vi "FTW-Message-Request-Interpret.vi"(8 "error in":errorcluster, 11 "FTW Incoming Request":refnum<class "FTW-Message-IncomingRequest.lvclass">) -> (0 "error out":errorcluster, 1 "Request Body":string, 2 "Request Header":string, 3 "FTW Incoming Request out":refnum<class "FTW-Message-IncomingRequest.lvclass">, 4 "Request Metadata":string)   [LabVIEW 2013, in "FTW-Message-IncomingRequest.lvclass"]
uses:
  FTW-Message-IncomingRequest.lvclass
  Base/FTW-Message.lvclass
panel:
  # "Inputs"
  # "Outputs"
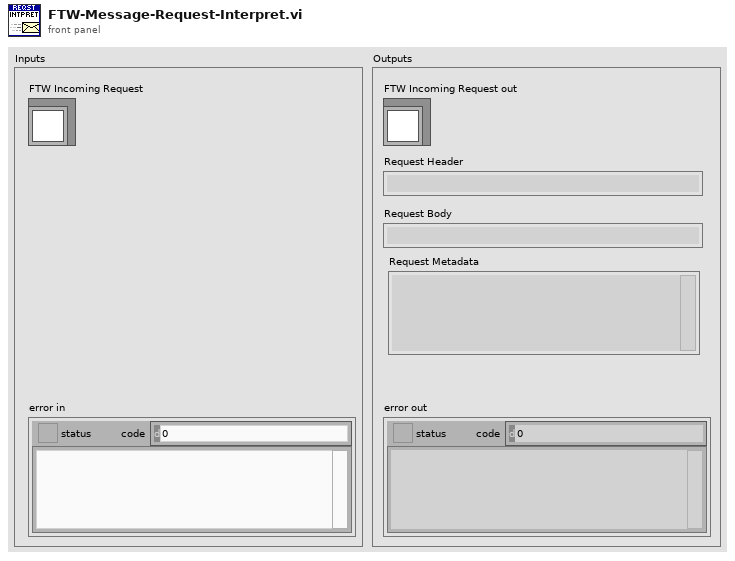
[diagram p1: front panel]
types:
  T1 = typedef "FTW-MessagePayload.ctl" = cluster{"Header":string, "Body":string, "Metadata":string}
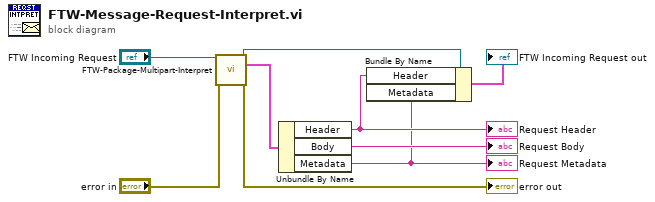
[diagram p0: block diagram]
diagram:
  n1 = call-dynamic "FTW-Package-Multipart-Interpret.vi"("FTW Message"="FTW Incoming Request", "error in"="error in") -> ("FTW Message out"=w8:refnum<class "FTW-Package.lvclass">, "Message"=w4:T1, "error out"=→"error out":errorcluster)  [unwired: 11 in]
  n2 = Unbundle By Name(w4) -> ("Header"=w2:string, "Body"=→"Request Body":string, "Metadata"=w1:string)
  "Request Header" <- w2
  "Request Metadata" <- w1
  n3 = Bundle By Name(cluster=w8, "Header"=w2, "Metadata"=w1) -> (→"FTW Incoming Request out":cluster{})
